vi "Temperature Monitor.vi"() -> ()   [LabVIEW 2015]
panel:
  out "Temperature History":cluster{dbl, "Temp":dbl}(graph)
  in  "Power":bool=TRUE
  # "On"
  # "Off"
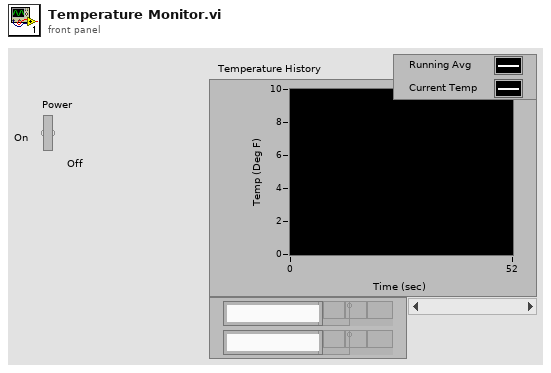
[diagram p1: front panel]
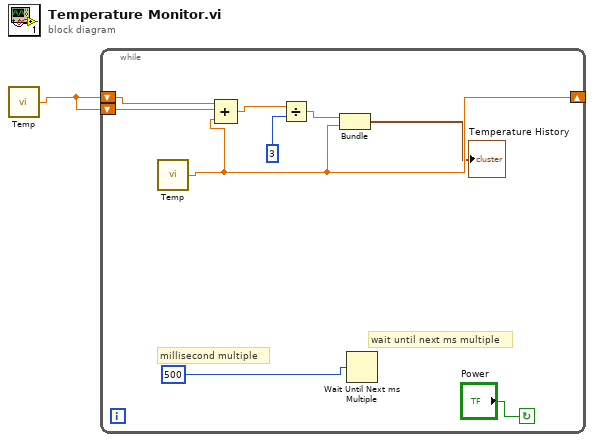
[diagram p0: block diagram]
diagram:
  n1 = call "Temp.vi"() -> ("Temp"=w1:dbl)  [unwired: 2 in]
  n2 = while {
    shift-right: [w3] -> _
    shift-left: w1 -> [w8]
    shift-left: w1 -> [w7]
    stop <- "Power" continue-if-true
    # "wait until next ms multiple"
    # "millisecond multiple"
    n3 = call "Temp.vi"() -> ("Temp"=w3:dbl)  [unwired: 2 in]
    n4 = Compound Arithmetic op=ADD(w8, w7, w3) -> (w5:dbl)
    n5 = Divide(x=w5, y=3) -> (x/y=w4:dbl)
    n6 = Bundle(w4, "Temp"=w3) -> (→"Temperature History":cluster{dbl, "Temp":dbl})  [unwired: 1 in]
    n7 = Wait Until Next ms Multiple(millisecond multiple=500) -> ()  [unwired: 1 out]
  }
